vi "Configure Report Generator.vi"(8 "error in (no error)":errorcluster, 11 "Report Generator In":refnum<class "Report Generator.lvclass">) -> (0 "error out":errorcluster, 3 "Report Generator Out":refnum<class "Report Generator.lvclass">)   [LabVIEW 2020, in "Reports.lvlib" / "Report Generator.lvclass"]
uses:
  Report Generator.lvclass
  C:/git/astemes-lunit/source/User Interface/Process/Process.lvclass
  User Interface/Process/Process.lvclass/Process.ctl
  User Interface/Process/Protected/Messaging/Enqueue Message.vi
  User Interface/Configuration Manager/Configuration Manager.lvclass
  Support/Utilities.lvlib
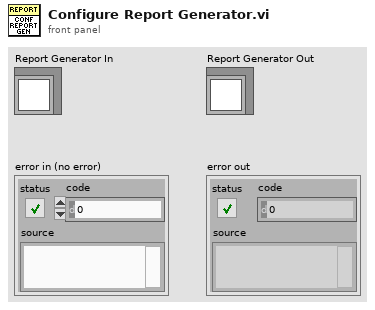
[diagram p1: front panel]
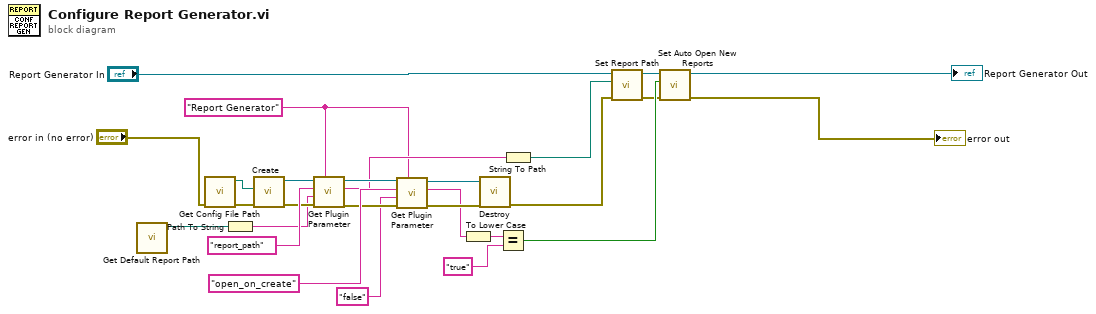
[diagram p0: block diagram]
diagram:
  w1 = "Report Generator"
  n1 = call "Get Default Report Path.vi"() -> ("Default Report Path"=w3:path)  [unwired: 10 in, 1 out]
  n2 = call "Get Config File Path.vi"("error in (no error)"="error in (no error)") -> ("error out"=w9:errorcluster, "Config Directory"=w13:path)  [unwired: 9 in]
  n3 = Path To String(path=w3) -> (string=w2:string)
  n4 = call "Create.vi"("error in (no error)"=w9, "configuration file path"=w13) -> ("error out"=w11:errorcluster, "Configuration Manager out"=w10:refnum<class "Configuration Manager.lvclass">)  [unwired: 8 in]
  n5 = call "Get Plugin Parameter.vi"("Plugin"=w1, "error in (no error)"=w11, "Default Value"=w2, "Name"="report_path", "Configuration Manager in"=w10) -> ("error out"=w12:errorcluster, "Value"=w14:string, "Configuration Manager out"=w19:refnum<class "Configuration Manager.lvclass">)  [unwired: 4 in]
  n6 = call "Get Plugin Parameter.vi"("Plugin"=w1, "error in (no error)"=w12, "Default Value"="false", "Name"="open_on_create", "Configuration Manager in"=w19) -> ("error out"=w18:errorcluster, "Value"=w5:string, "Configuration Manager out"=w20:refnum<class "Configuration Manager.lvclass">)  [unwired: 4 in]
  n7 = To Lower Case(string=w5) -> (all lower case string=w23:string)
  n8 = call "Destroy.vi"("error in (no error)"=w18, "Configuration Manager In"=w20) -> ("error out"=w6:errorcluster)  [unwired: 9 in]
  n9 = Equal?(x=w23, y="true") -> (x = y?=w25:bool)
  n10 = String To Path(string=w14) -> (path=w16:path)
  n11 = call "Set Report Path.vi"("error in (no error)"=w6, "Report Directory"=w16, "Report Generator In"="Report Generator In") -> ("error out"=w8:errorcluster, "Report Generator Out"=w17:refnum<class "Report Generator.lvclass">)  [unwired: 7 in]
  n12 = call "Set Auto Open New Reports.vi"("error in (no error)"=w8, "Open New Reports?"=w25, "Report Generator In"=w17) -> ("error out"=→"error out":errorcluster, "Report Generator Out"=→"Report Generator Out":refnum<class "Report Generator.lvclass">)  [unwired: 7 in]
